vi "UIDisable.vi"(8 "error in (no error)":errorcluster, 10 "UI":T1, 11 "Status:":refnum<vi>) -> (0 "error out":errorcluster)   [LabVIEW 2009]
uses:
  Global Variables.vi
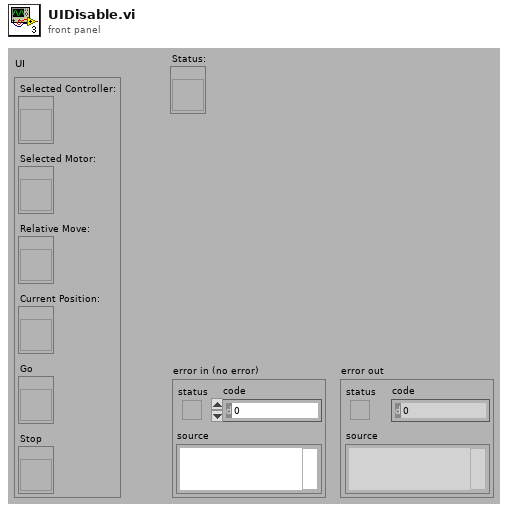
[diagram p1: front panel]
types:
  T1 = cluster{"Selected Controller:":refnum<vi>, "Selected Motor:":refnum<vi>, "Relative Move:":refnum<vi>, "Current Position:":refnum<vi>, "Go":refnum<vi>, "Stop":refnum<vi>}
  T2 = enum8{"Enabled", "Disabled", "Disabled and Grayed Out"}
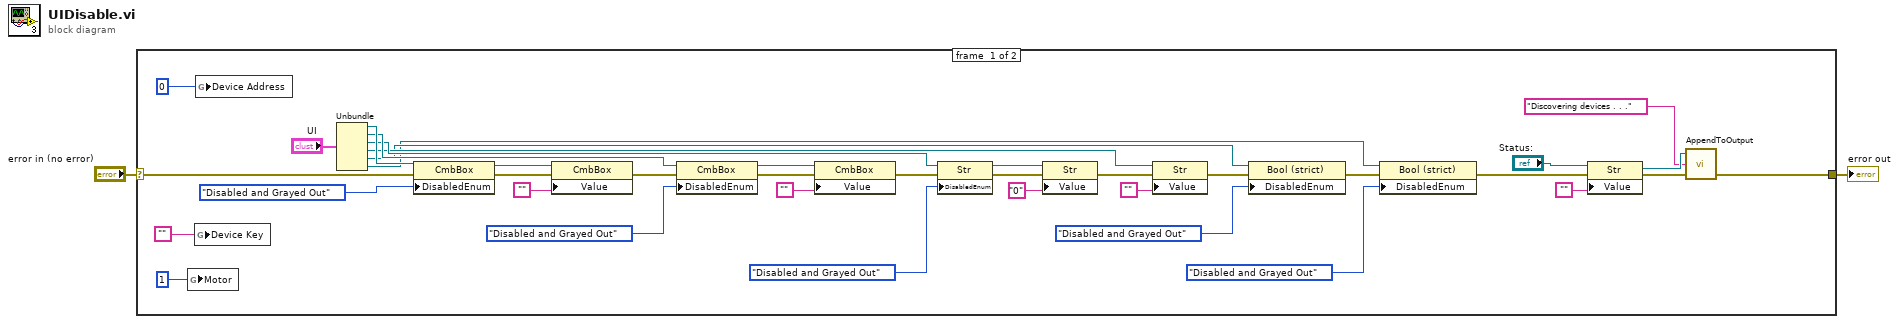
[diagram p0: block diagram]
diagram:
  n1 = case shown="No Error" "error in (no error)" {
    selector: "error in (no error)" -> [w33 w41]
    tunnel: [w23 w41] -> w1
    frame #0 {
      n2 = global write "Global Variables.vi" "Motor"(1 ("Motor")) -> ()
      n3 = global write "Global Variables.vi" "Device Key"("") -> ()
      n4 = global write "Global Variables.vi" "Device Address"(0 ("Device Address")) -> ()
      n5 = Unbundle("UI") -> ("Selected Controller:"=w9:refnum<vi>, "Selected Motor:"=w8:refnum<vi>, "Relative Move:"=w7:refnum<vi>, "Current Position:"=w6:refnum<vi>, "Go"=w5:refnum<vi>, "Stop"=w4:refnum<vi>)
      n6 = property on="Property Node" class="CmbBox"(reference=w9, error in=w33, "DisabledEnum"=T2."Disabled and Grayed Out" ("Disabled")) -> (reference out=w32:refnum<vi>, error out=w28:errorcluster)
      n7 = property class="CmbBox"(reference=w32, error in=w28, "Value"="") -> (error out=w27:errorcluster)  [unwired: 1 out]
      n8 = property on="Property Node" class="CmbBox"(reference=w8, error in=w27, "DisabledEnum"=T2."Disabled and Grayed Out" ("Disabled")) -> (reference out=w30:refnum<vi>, error out=w26:errorcluster)
      n9 = property class="CmbBox"(reference=w30, error in=w26, "Value"="") -> (error out=w25:errorcluster)  [unwired: 1 out]
      n10 = property on="Property Node" class="Str"(reference=w7, error in=w25, "DisabledEnum"=T2."Disabled and Grayed Out" ("Disabled")) -> (reference out=w17:refnum<vi>, error out=w18:errorcluster)
      n11 = property class="Str"(reference=w17, error in=w18, "Value"="0") -> (error out=w15:errorcluster)  [unwired: 1 out]
      n12 = property on="Property Node" class="Str"(reference=w6, error in=w15, "Value"="") -> (error out=w14:errorcluster)  [unwired: 1 out]
      n13 = property on="Property Node" class="Bool (strict)"(reference=w5, error in=w14, "DisabledEnum"=T2."Disabled and Grayed Out" ("Disabled")) -> (error out=w35:errorcluster)  [unwired: 1 out]
      n14 = property on="Property Node" class="Bool (strict)"(reference=w4, error in=w35, "DisabledEnum"=T2."Disabled and Grayed Out" ("Disabled")) -> (error out=w3:errorcluster)  [unwired: 1 out]
      n15 = property class="Str"(reference="Status:", error in=w3, "Value"="") -> (reference out=w24:refnum<vi>, error out=w22:errorcluster)
      n16 = call "AppendToOutput.vi"("error in"=w22, "Input String"="Discovering devices . . .", "Output Refnum In"=w24) -> ("error out"=w23:errorcluster)  [unwired: 1 in, 1 out]
    }
    frame #1 {
    }
  }
  "error out" <- w1
